vi "获取奶茶清单.vi"(7 "父类":string, 8 "error in (no error)":errorcluster caption="错误输入（无错误）", 9 "Folder Path":path caption="文件夹路径", 11 "奶茶 输入":refnum<class "奶茶.lvclass">) -> (0 "error out":errorcluster caption="错误输出", 1 "清单名称":string[](array[string]), 2 "数组":refnum<class>[](array[class]), 3 "奶茶 输出":refnum<class "奶茶.lvclass">)   [LabVIEW 2016, in "奶茶.lvclass"]
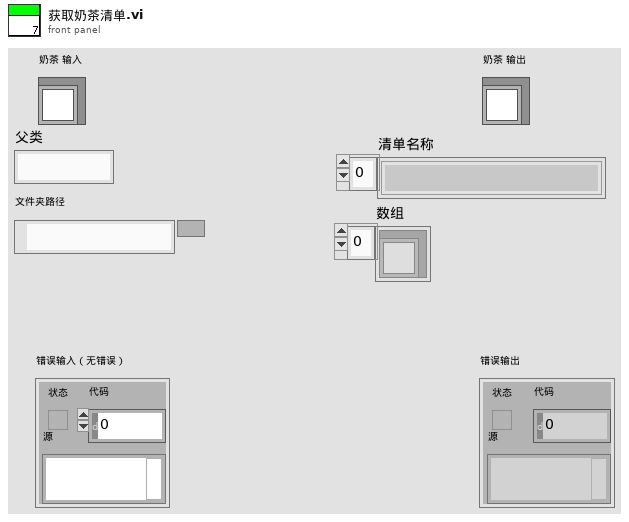
[diagram p1: front panel]
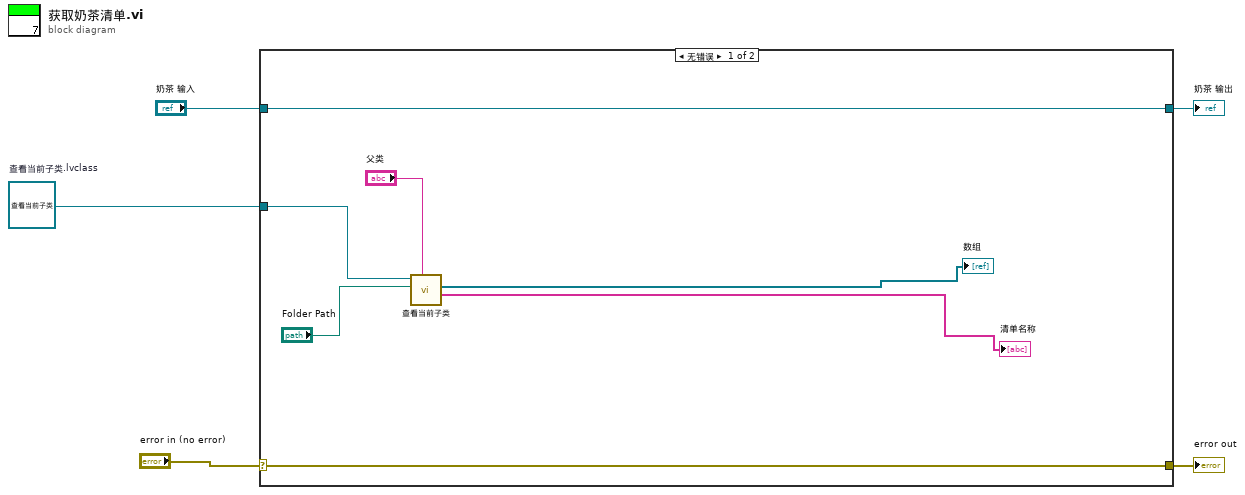
[diagram p0: block diagram]
diagram:
  w1 = refnum<class "查看当前子类.lvclass"> refnum  # 查看当前子类.lvclass
  n1 = case shown="无错误" "error in (no error)" {
    selector: "error in (no error)" -> [w12 w14]
    tunnel: [w12 w14] -> w4
    tunnel: [w11 w13] -> w2
    tunnel: "奶茶 输入" -> [w11 w13]
    tunnel: w1 -> [w10 _]
    frame No Error {
      n2 = call-dynamic "查看当前子类.vi"("父类"="父类", "Folder Path"="Folder Path", "查看当前子类 输入"=w10) -> ("清单名称"=→"清单名称":string[], "数组"=→"数组":refnum<class>[])  [unwired: 5 in, 2 out]
    }
    frame Error {
    }
  }
  "error out" <- w4
  "奶茶 输出" <- w2
